vi "Channel Group Page.vi"(8 "error in (no error)":errorcluster, 11 "Node Ptr":T1 format="%.0x") -> (0 "error out":errorcluster)   [LabVIEW 2027, in "Embedded Data Logger System Explorer.lvlib"]
uses:
  Embedded Data Logger System Explorer.lvlib
  <vilib>/NI VeriStand/Custom Device API/Custom Device API.lvlib
  <vilib>/NI VeriStand/Custom Device API/Custom Device Item Ref.ctl
  <vilib>/Utility/miscctls.llb/LVRowAndColumnUnsignedTypeDef.ctl
  <vilib>/NI VeriStand/Custom Device API/Get Item Property (Boolean).vi
  <vilib>/NI VeriStand/Custom Device Tools/Custom Device Utility Library/Custom Device Utility Library.lvlib
  Scripting/Embedded Data Logger Scripting.lvlib
panel:
  in  "Logged Channels":i32[](listbox)
  in  "Remove":bool
  in  "Add Channels":bool
  in  "Header":cluster{"Section Name":string}={"Section Name"="Channel Group Settings"}
  in  "Description":string
  in  "Name":string
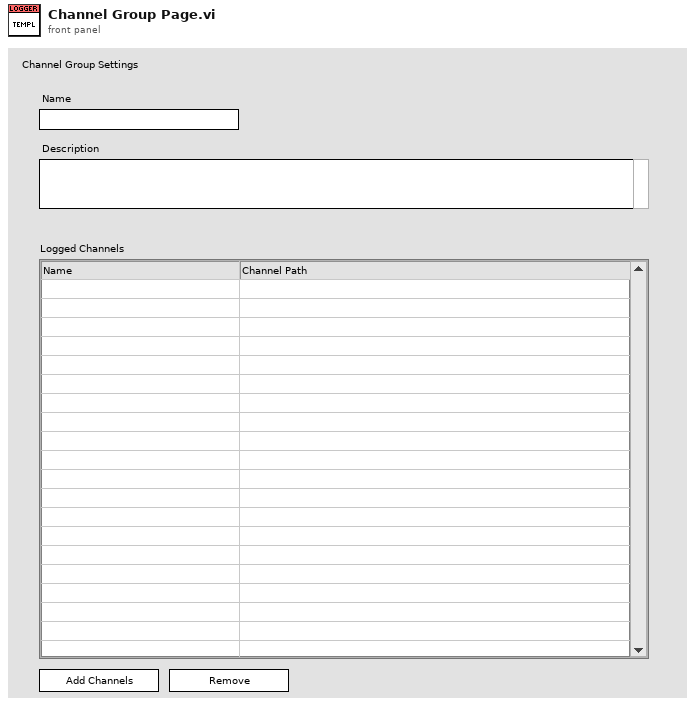
[diagram p1: front panel]
types:
  T1 = typedef "Custom Device API.lvlib/Custom Device Item Ref.ctl" = u64
  T2 = typedef "Custom Device API.lvlib/Custom Device Item Info.ctl" = cluster{"Name":string, "Is Channel":bool, "GUID":string, "Is Waveform":bool}
  T3 = typedef "LVRowAndColumnUnsignedTypeDef.ctl" = cluster{"Row":u32, "Column":u32}
  T4 = typedef "Custom Device API.lvlib/Custom Device Commands.ctl" = enum16{"Default", "Item renamed", "Shutdown", "Dynamic button pressed"}
  T5 = typedef "LVRowAndColumnTypeDef.ctl" = cluster{"Row":i32, "Column":i32}
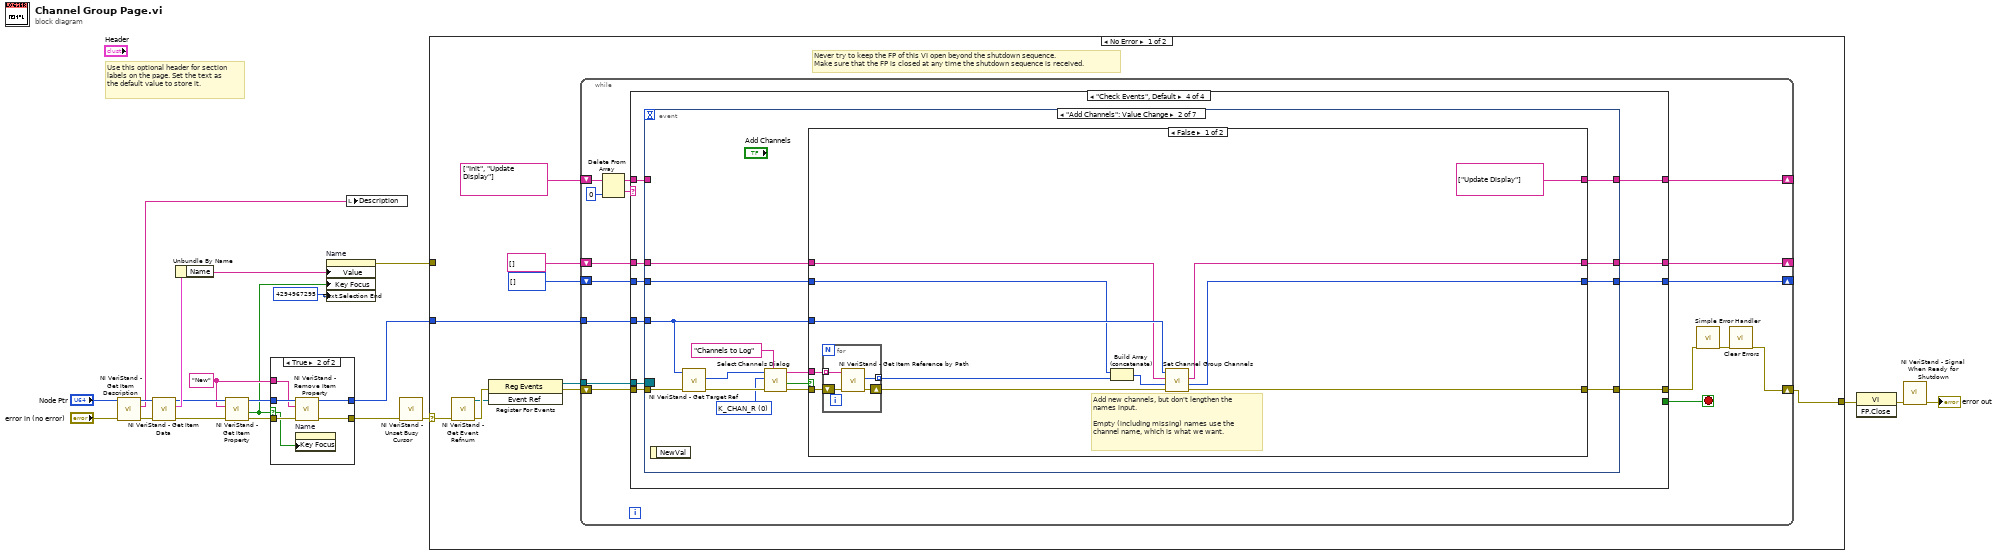
[diagram p0: block diagram]
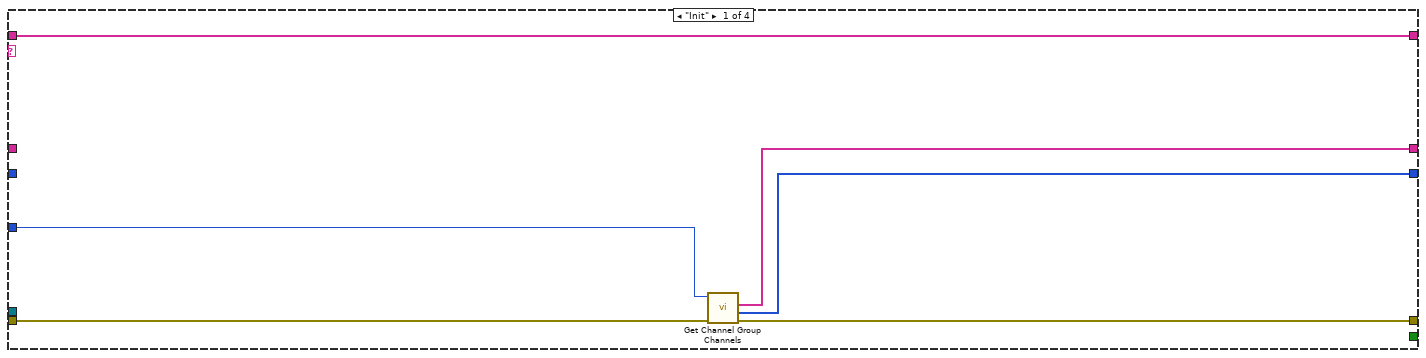
[diagram p3: hidden frame]
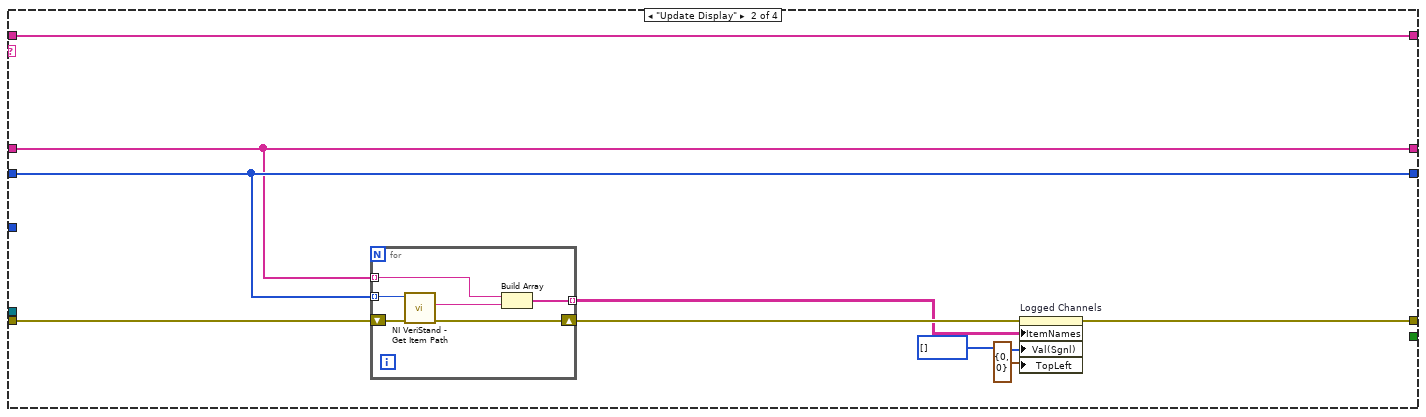
[diagram p4: hidden frame]
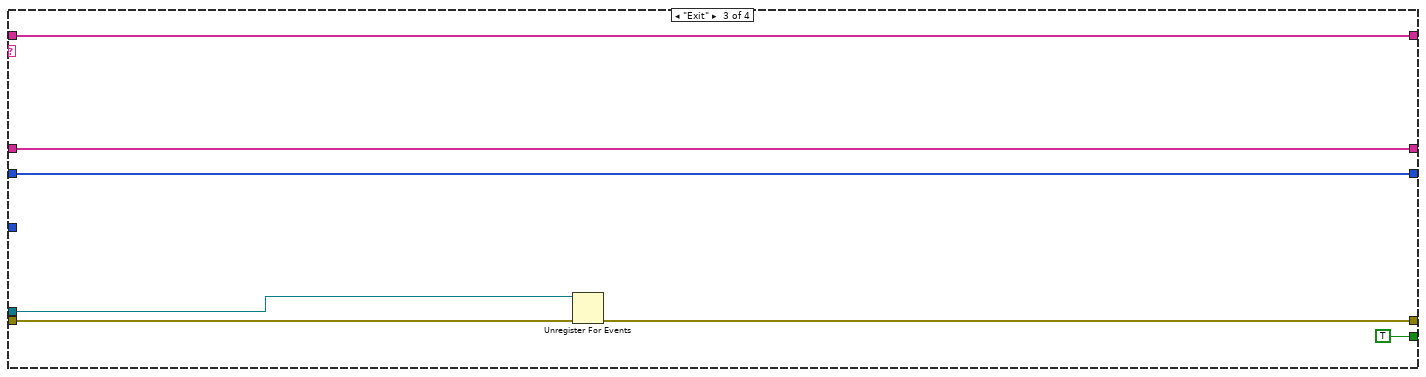
[diagram p5: hidden frame]
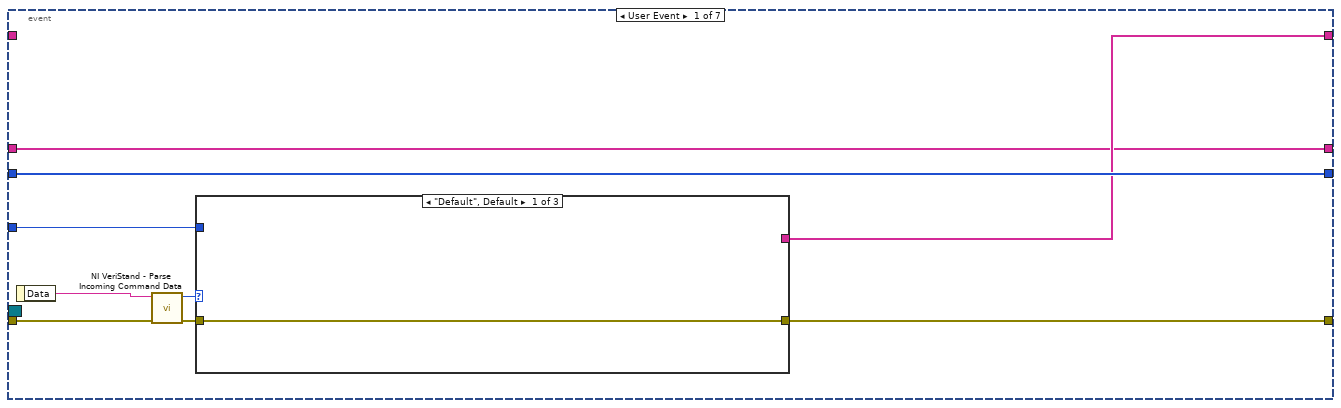
[diagram p6: hidden frame]
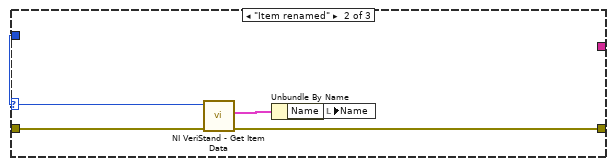
[diagram p7: hidden frame]
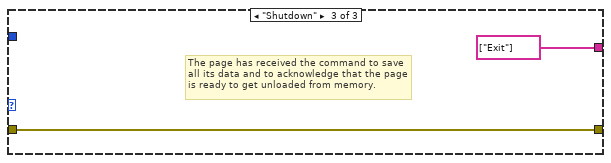
[diagram p8: hidden frame]
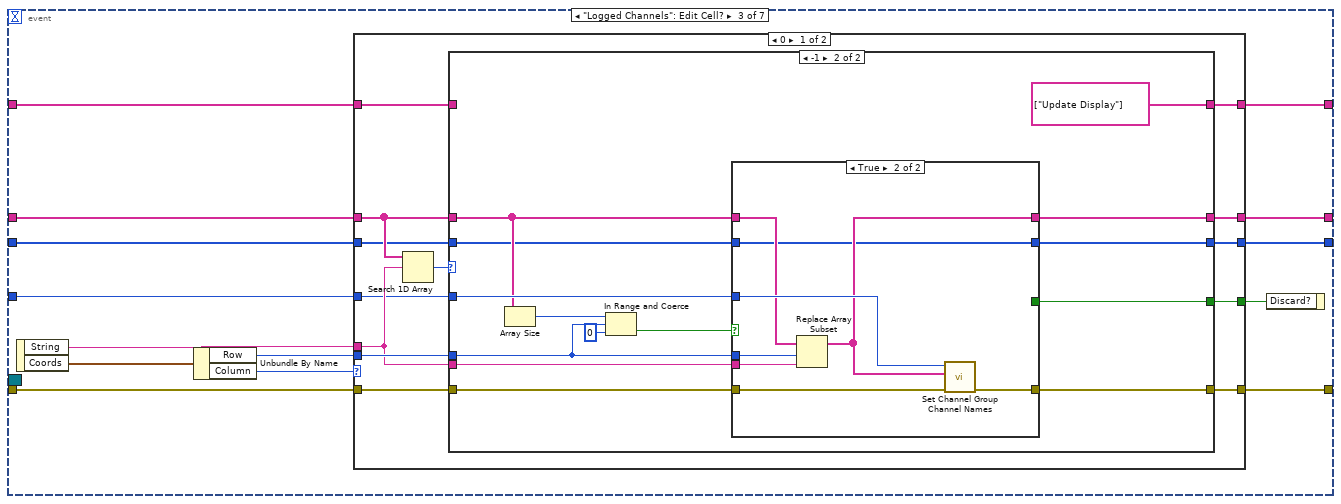
[diagram p10: hidden frame]
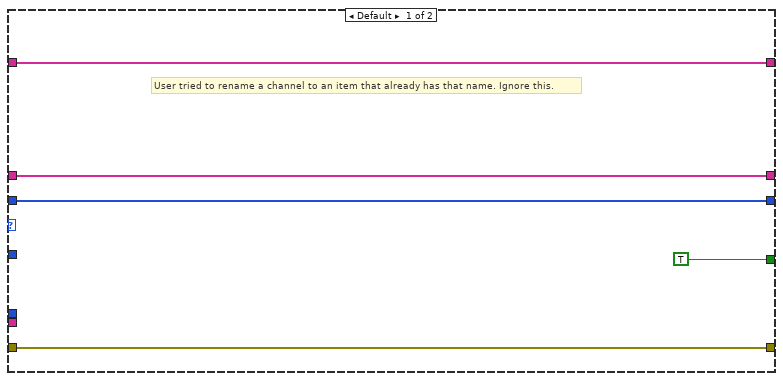
[diagram p11: hidden frame]
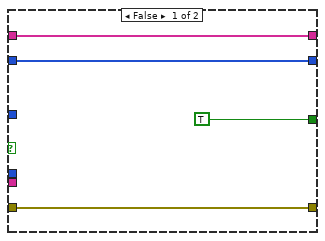
[diagram p12: hidden frame]
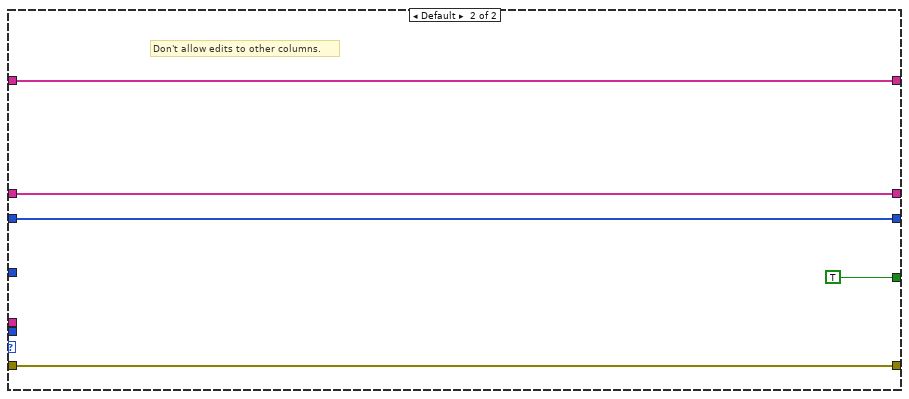
[diagram p13: hidden frame]
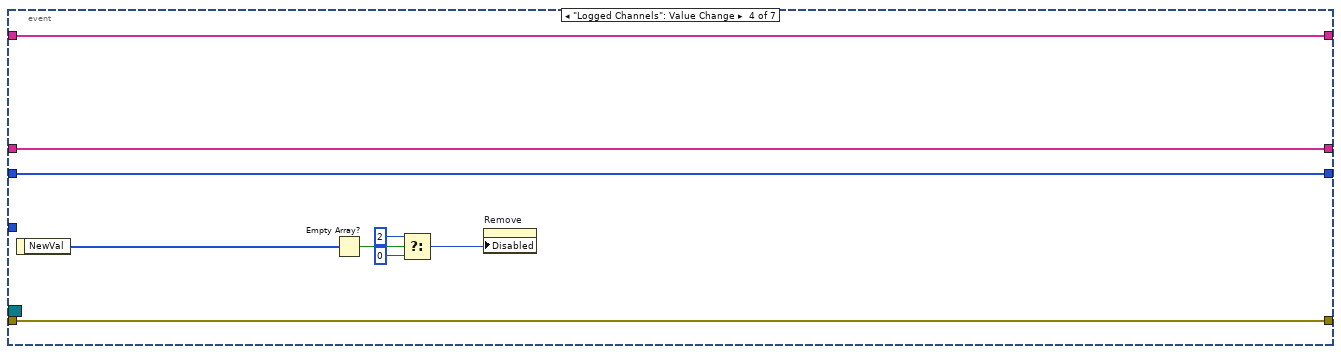
[diagram p14: hidden frame]
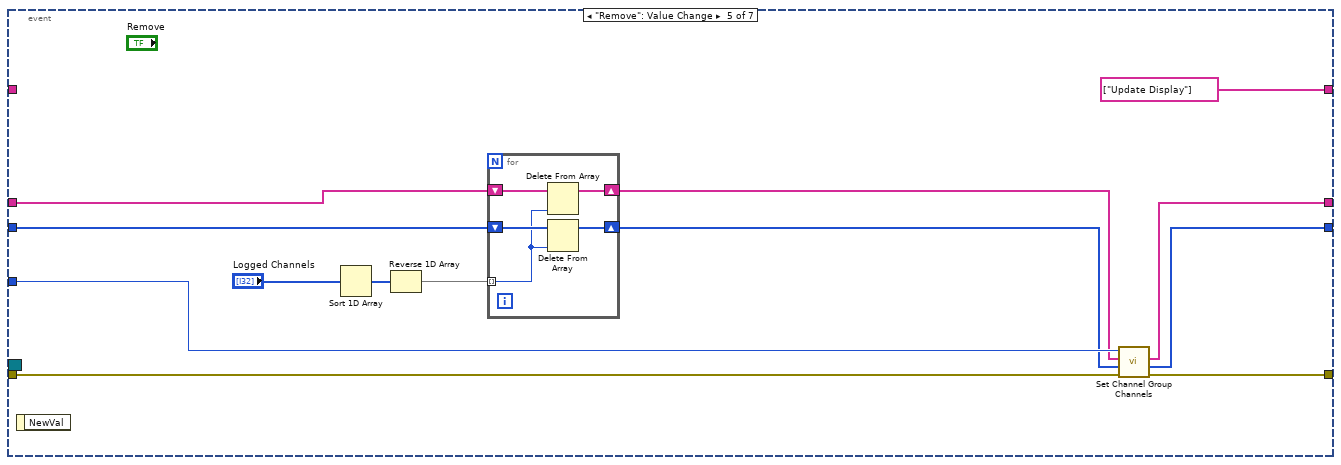
[diagram p15: hidden frame]
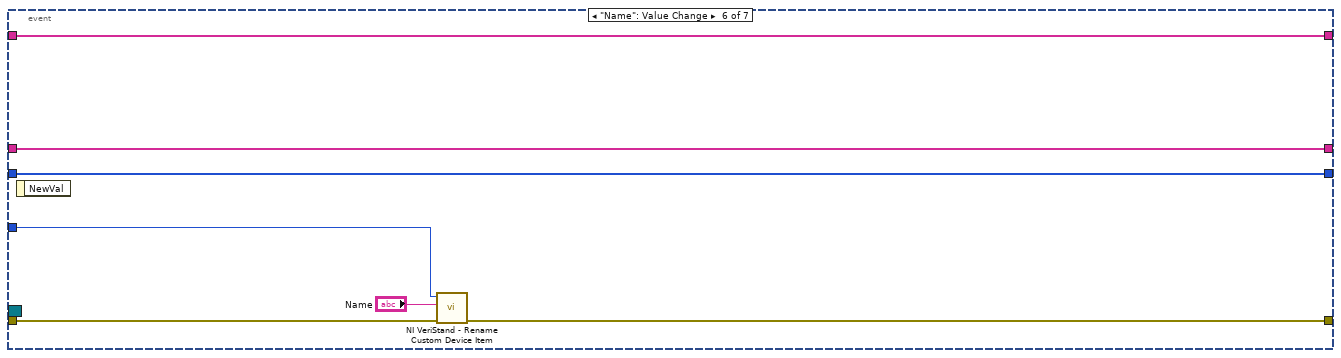
[diagram p16: hidden frame]
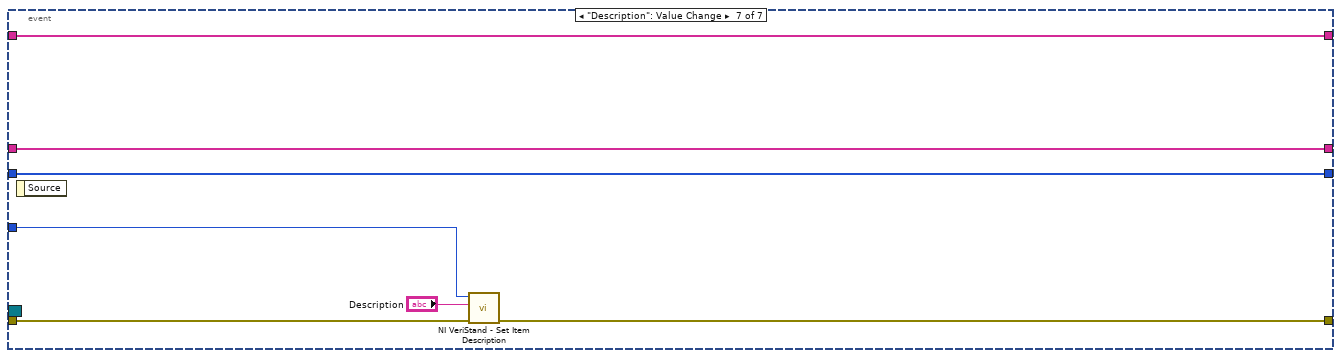
[diagram p17: hidden frame]
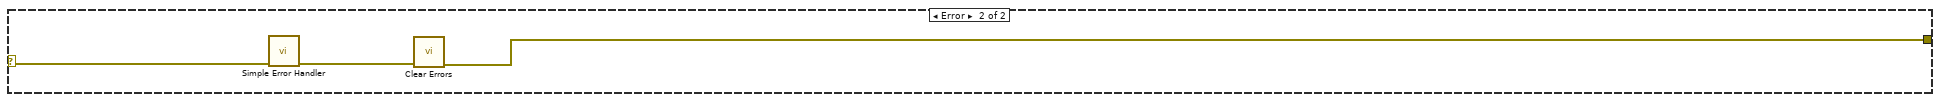
[diagram p18: hidden frame]
diagram:
  w5 = "New" ("Property Name")
  # "Use this optional header for section labels on the page. Set the text as the default value to store it."
  n1 = call <vilib>:"NI VeriStand - Get Item Description.vi"("error in (no error)"="error in (no error)", "Item Ref in"="Node Ptr") -> ("error out"=w13:errorcluster, "Description"=w14:string, "Item Ref out"=w15:T1)  [unwired: 7 out]
  n2 = call <vilib>:"NI VeriStand - Get Item Data.vi"("error in (no error)"=w13, "Item Ref in"=w15) -> ("error out"=w11:errorcluster, "Item Info"=w12:T2, "Item Ref out"=w10:T1)  [unwired: 7 out]
  n3 = Unbundle By Name(w12) -> ("Name"=w3:string)
  n4 = call-poly <vilib>:"NI VeriStand - Get Item Property.vi"("error in (no error)"=w11, "Property Name"=w5, "Item Ref in"=w10) -> ("error out"=w9:errorcluster, "Value"=w2:bool, "Item Ref out"=w7:T1)  [unwired: 5 in, 1 out]
  n5 = case shown="True" w2 {
    selector: w2 -> [_ w24]
    tunnel: w9 -> [w23 w28]
    tunnel: [w23 w25] -> w8
    tunnel: w7 -> [w22 w29]
    tunnel: [w22 w26] -> w6
    tunnel: w5 -> [_ w27]
    frame False {
    }
    frame True {
      n6 = property on="Name" class="Str"("Key Focus"=w24) -> ()  [unwired: 2 in, 2 out]
      n7 = call <vilib>:"NI VeriStand - Remove Item Property.vi"("error in (no error)"=w28, "Property Name"=w27, "Item Ref in"=w29) -> ("error out"=w25:errorcluster, "Item Ref out"=w26:T1)  [unwired: 6 in, 1 out]
    }
  }
  n8 = property on="Name" class="Str"("Value"=w3, "Key Focus"=w2, "Text.Selection End"=u32 4294967295 ("Text.Selection:End")) -> (error out=w1:errorcluster)  [unwired: 2 in, 1 out]
  n9 = local write "Description"(w14) -> ()
  n10 = call <vilib>:"NI VeriStand - Unset Busy Cursor.vi"("error in (no error)"=w8) -> ("error out"=w17:errorcluster)  [unwired: 10 out]
  n11 = case shown="No Error" w17 {
    selector: w17 -> [w34 w251]
    tunnel: [w31 w249] -> w21
    tunnel: w6 -> [w36 _]
    tunnel: w1 -> [_ _]
    frame No Error {
      # "Never try to keep the FP of this VI open beyond the shutdown sequence.\nMake sure that the FP is closed at any time the shutdown sequence is received."
      n12 = call <vilib>:"NI VeriStand - Get Event Refnum.vi"("error in (no error)"=w34) -> ("error out"=w39:errorcluster, "Event Ref"=w38:refnum<user-event>)  [unwired: 9 out]
      n13 = register-events(error in=w39, w38) -> (reference out=w32:refnum<event-registration>, error out=w37:errorcluster)  [unwired: 1 in]
      n14 = while {
        tunnel: w36 -> [w53]
        shift-right: [w50] -> w31
        shift-left: w37 -> [w55]
        shift-right: [w48] -> _
        shift-left: T1[] [] ("Selected Channel Refs") -> [w49]
        shift-right: [w44] -> _
        shift-left: string[] ["Init", "Update Display"] -> [w47]
        tunnel: w32 -> [w42]
        shift-right: [w40] -> _
        shift-left: string[] [] -> [w41]
        stop <- w54 stop-if-true
        n15 = Delete From Array(array=w47, index=0) -> (deleted portion=w43:string, array with subset deleted=w45:string[])  [unwired: 1 in]
        n16 = case shown="\"Check Events\", Default" w43 {
          tunnel: w55 -> [w60 w70 w80 w93]
          tunnel: w42 -> [_ _ w78 w92]
          tunnel: [_ _ TRUE _] -> w54
          tunnel: w53 -> [w59 _ _ w91]
          tunnel: [w58 w62 w79 w90] -> w52
          tunnel: w49 -> [_ w69 w83 w89]
          tunnel: [w56 w69 w83 w88] -> w48
          tunnel: w45 -> [w61 w66 w82 w87]
          tunnel: [w61 w66 w82 w86] -> w44
          tunnel: w41 -> [_ w63 w77 w85]
          tunnel: [w57 w63 w77 w84] -> w40
          frame "Init" {
            n17 = call "Get Channel Group Channels.vi"("error in"=w60, "channel group in"=w59) -> ("error out"=w58:errorcluster, "channels"=w56:T1[], "names"=w57:string[])  [unwired: 6 in, 1 out]
          }
          frame "Update Display" {
            n18 = for {
              shift-right: [w74] -> w68
              shift-left: w70 -> [w76]
              tunnel: w69 -> [w75] mode=indexing
              tunnel: [w72] -> w67 mode=indexing
              tunnel: w63 -> [w71] mode=indexing
              n19 = call <vilib>:"NI VeriStand - Get Item Path.vi"("error in (no error)"=w76, "Item Ref in"=w75) -> ("error out"=w74:errorcluster, "Path"=w73:string)  [unwired: 8 out]
              n20 = Build Array(w71, w73) -> (w72:string[])
            }
            n21 = property on="Logged Channels" class="MCListbox (strict)"(error in=w68, "ItemNames"=w67, "Val(Sgnl)"=i32[] [] ("Value (Signaling)"), "TopLeft"=T3 {"Row"=0, "Column"=0} ("Top Left Visible Cell")) -> (error out=w62:errorcluster)  [unwired: 1 in, 1 out]
          }
          frame "Exit" {
            n22 = Unregister For Events(event registration refnum=w78, error in=w80) -> (error out=w79:errorcluster)
          }
          frame "Check Events", Default {
            n23 = event shown="[1] \"Add Channels\": Value Change" {
              selector: w92 -> [_ _ _ _ _ _ _]
              dyn-events: _ -> [_ _ _ _ _ _ _]
              timeout: _ -> [_ _ _ _ _ _ _]
              tunnel: w93 -> [w102 w115 w147 w210 w223 w241 w247]
              tunnel: [w98 w120 w145 w210 w222 w240 w246] -> w90
              tunnel: w91 -> [w97 w116 w146 _ w221 w239 w248]
              tunnel: w89 -> [w96 w125 w157 w216 w228 w237 w244]
              tunnel: [w96 w121 w154 w216 w218 w237 w244] -> w88
              tunnel: w87 -> [_ _ w149 w215 _ w236 w243]
              tunnel: [w95 w119 w148 w215 string[] ["Update Display"] w236 w243] -> w86
              tunnel: w85 -> [w94 w118 w156 w208 w224 w235 w242]
              tunnel: [w94 w117 w155 w208 w219 w235 w242] -> w84
              event User Event {
                n24 = event-data() -> ("Data"=w101:string)  [unwired: 1 out]
                n25 = call <vilib>:"NI VeriStand - Parse Incoming Command Data.vi"("error in (no error)"=w102, "Incoming data"=w101) -> ("error out"=w100:errorcluster, "Action"=w99:T4)  [unwired: 8 out]
                n26 = case shown="\"Default\", Default" w99 {
                  tunnel: w100 -> [w103 w108 w110]
                  tunnel: [w103 w105 w110] -> w98
                  tunnel: w97 -> [_ w107 _]
                  tunnel: [_ _ string[] ["Exit"]] -> w95
                  frame "Default", Default {
                  }
                  frame "Item renamed" {
                    n27 = call <vilib>:"NI VeriStand - Get Item Data.vi"("error in (no error)"=w108, "Item Ref in"=w107) -> ("error out"=w105:errorcluster, "Item Info"=w106:T2)  [unwired: 8 out]
                    n28 = Unbundle By Name(w106) -> ("Name"=w104:string)
                    n29 = local write "Name"(w104) -> ()
                  }
                  frame "Shutdown" {
                    # "The page has received the command to save all its data and to acknowledge that the page is ready to get unloaded from memory."
                  }
                }
              }
              event "Add Channels": Value Change {
                w111 = u8 0 items=["K_CHAN_R", "K_CHAN_W", "K_CHAN_RW", "K_CHAN_VOLT", "K_CHAN_FAULT", "K_ALL", "K_CUSTOM"] ("Filter")
                n30 = event-data() -> ()  [unwired: 2 out]
                n31 = call <vilib>:"NI VeriStand - Get Target Ref.vi"("error in"=w115, "Item Ref in"=w116) -> ("error out"=w114:errorcluster, "Target Ref"=w113:T1)  [unwired: 6 in, 2 out]
                n32 = call "Select Channels Dialog.vi"("Channel Label"="Channels to Log", "error in (no error)"=w114, "Filter"=w111, "Start Item Ref"=w113) -> ("error out"=w124:errorcluster, "Canceled"=w123:bool, "Channels"=w122:string[])  [unwired: 2 in, 3 out]
                n33 = case shown="False" w123 {
                  tunnel: w125 -> [w129 w144]
                  tunnel: w124 -> [w136 w143]
                  tunnel: w122 -> [w135 _]
                  tunnel: [w130 w144] -> w121
                  tunnel: [w132 w143] -> w120
                  tunnel: w116 -> [w133 _]
                  tunnel: [string[] ["Update Display"] _] -> w119
                  tunnel: w118 -> [w126 w142]
                  tunnel: [w131 w142] -> w117
                  frame False {
                    # "Add new channels, but don't lengthen the names input.\n\nEmpty (including missing) names use the channel name, which is what we want."
                    n34 = for {
                      shift-right: [w140] -> w134
                      shift-left: w136 -> [w141]
                      tunnel: w135 -> [w139] mode=indexing
                      tunnel: [w138] -> w128 mode=indexing
                      n35 = call <vilib>:"NI VeriStand - Get Item Reference by Path.vi"("error in (no error)"=w141, "Item Path in"=w139) -> ("error out"=w140:errorcluster, "Item Ref"=w138:T1)  [unwired: 6 in, 2 out]
                    }
                    n36 = Build Array (concatenate)(w129, w128) -> (w127:T1[])
                    n37 = call "Set Channel Group Channels.vi"("error in"=w134, "channels"=w127, "names"=w126, "channel group in"=w133) -> ("error out"=w132:errorcluster, "saved channels"=w130:T1[], "saved names"=w131:string[])  [unwired: 4 in, 1 out]
                  }
                  frame True {
                    # "User canceled out of the dialog."
                  }
                }
              }
              event "Logged Channels": Edit Cell? {
                n38 = event-data() -> ("String"=w150:string, "Coords"=w158:T5)  [unwired: 1 out]
                n39 = Unbundle By Name(w158) -> ("Row"=w152:i32, "Column"=w153:i32)
                n40 = case shown="0" w153 {
                  tunnel: w157 -> [w164 w206]
                  tunnel: w156 -> [w166 w207]
                  tunnel: [w167 w207] -> w155
                  tunnel: [w165 w206] -> w154
                  tunnel: w152 -> [w163 _]
                  tunnel: [w170 TRUE] -> w151
                  tunnel: w150 -> [w162 _]
                  tunnel: w149 -> [w168 w204]
                  tunnel: [w169 w204] -> w148
                  tunnel: w147 -> [w161 w203]
                  tunnel: w146 -> [w160 _]
                  tunnel: [w159 w203] -> w145
                  frame 0 {
                    n41 = Search 1D Array(1D array=w166, element=w162) -> (index of element=w171:i32)  [unwired: 1 in]
                    n42 = case shown="-1" w171 {
                      tunnel: [TRUE w177] -> w170
                      tunnel: [w175 string[] ["Update Display"]] -> w169
                      tunnel: w168 -> [w175 _]
                      tunnel: [w174 w186] -> w167
                      tunnel: w166 -> [w174 w184]
                      tunnel: [w173 w183] -> w165
                      tunnel: w164 -> [w173 w182]
                      tunnel: w163 -> [_ w180]
                      tunnel: w162 -> [_ w189]
                      tunnel: w161 -> [w172 w188]
                      tunnel: w160 -> [_ w187]
                      tunnel: [w172 w185] -> w159
                      frame Default {
                        # "User tried to rename a channel to an item that already has that name. Ignore this."
                      }
                      frame -1 {
                        n43 = Array Size(array=w184) -> (size(s)=w181:i32)
                        n44 = In Range and Coerce(upper limit=w181, x=w180, lower limit=0) -> (In Range?=w179:bool)  [unwired: 1 out]
                        n45 = case shown="True" w179 {
                          tunnel: w180 -> [_ w202]
                          tunnel: w189 -> [_ w201]
                          tunnel: w188 -> [w192 w200]
                          tunnel: w187 -> [_ w199]
                          tunnel: [w194 w198] -> w186
                          tunnel: [w192 w197] -> w185
                          tunnel: w184 -> [w194 w196]
                          tunnel: [w193 w195] -> w183
                          tunnel: w182 -> [w193 w195]
                          tunnel: [TRUE _] -> w177
                          frame False {
                          }
                          frame True {
                            n46 = Replace Array Subset(array=w196, new element=w201, index=w202) -> (w198:string[])
                            n47 = call "Set Channel Group Channel Names.vi"("error in (no error)"=w200, "names"=w198, "channel group in"=w199) -> ("error out"=w197:errorcluster)  [unwired: 7 in, 1 out]
                          }
                        }
                      }
                    }
                  }
                  frame Default {
                    # "Don't allow edits to other columns."
                  }
                }
                n48 = event-data("Discard?"=w151) -> ()  [unwired: 1 in, 1 out]
              }
              event "Logged Channels": Value Change {
                n49 = event-data() -> ("NewVal"=w209:i32[])  [unwired: 1 out]
                n50 = Empty Array?(array=w209) -> (empty?=w214:bool)
                n51 = Select(t=u8 2, s=w214, f=u8 0) -> (s? t:f=w211:u8)
                n52 = property on="Remove" class="Bool"("Disabled"=w211) -> ()  [unwired: 2 in, 2 out]
              }
              event "Remove": Value Change {
                n53 = event-data() -> ()  [unwired: 2 out]
                n54 = Sort 1D Array(array="Logged Channels") -> (sorted array=w229:i32[])
                n55 = Reverse 1D Array(array=w229) -> (reversed array=w227:i32[])
                n56 = for {
                  shift-right: [w233] -> w217
                  shift-left: w228 -> [w234]
                  tunnel: w227 -> [w230] mode=indexing
                  shift-right: [w231] -> w220
                  shift-left: w224 -> [w232]
                  n57 = Delete From Array(array=w232, index=w230) -> (array with subset deleted=w231:string[])  [unwired: 1 in, 1 out]
                  n58 = Delete From Array(array=w234, index=w230) -> (array with subset deleted=w233:T1[])  [unwired: 1 in, 1 out]
                }
                n59 = call "Set Channel Group Channels.vi"("error in"=w223, "channels"=w217, "names"=w220, "channel group in"=w221) -> ("error out"=w222:errorcluster, "saved channels"=w218:T1[], "saved names"=w219:string[])  [unwired: 4 in, 1 out]
              }
              event "Name": Value Change {
                n60 = event-data() -> ()  [unwired: 2 out]
                n61 = call <vilib>:"NI VeriStand - Rename Custom Device Item.vi"("error in (no error)"=w241, "New Name"="Name", "Item Ref in"=w239) -> ("error out"=w240:errorcluster)  [unwired: 1 in, 7 out]
              }
              event "Description": Value Change {
                n62 = event-data() -> ()  [unwired: 2 out]
                n63 = call <vilib>:"NI VeriStand - Set Item Description.vi"("error in (no error)"=w247, "Description"="Description", "Item Ref in"=w248) -> ("error out"=w246:errorcluster)  [unwired: 8 out]
              }
            }
          }
        }
        n64 = call <vilib>:"Simple Error Handler.vi"("error in (no error)"=w52) -> ("error out"=w51:errorcluster)  [unwired: 1 in, 7 out]
        n65 = call <vilib>:"Clear Errors.vi"("error in (no error)"=w51) -> ("error out"=w50:errorcluster)  [unwired: 1 in, 5 out]
      }
    }
    frame Error {
      n66 = call <vilib>:"Simple Error Handler.vi"("error in (no error)"=w251) -> ("error out"=w250:errorcluster)  [unwired: 1 in, 7 out]
      n67 = call <vilib>:"Clear Errors.vi"("error in (no error)"=w250) -> ("error out"=w249:errorcluster)  [unwired: 1 in, 5 out]
    }
  }
  n68 = invoke class="VI" method="FP.Close"(error in=w21) -> (error out=w20:errorcluster)  [unwired: 2 in, 2 out]
  n69 = call <vilib>:"NI VeriStand - Signal When Ready for Shutdown.vi"("error in (no error)"=w20) -> ("error out"=→"error out":errorcluster)  [unwired: 10 out]
